vi "Setup Power Supply.vi"(0 "reference in":refnum<class "Power Supply.lvclass">, 1 "Power Supply Chain VISA Session":refnum<visa-resource-name>, 4 "Power Supply Chain Address":i16, 5 "error in (no error)":errorcluster) -> (14 "reference out":refnum<class "Power Supply.lvclass">, 15 "Power Supply Chain VISA Session OUT":refnum<visa-resource-name>, 19 "error out":errorcluster)   [LabVIEW 2017, in "Power Supply.lvclass"]
uses:
  Power Supply.lvclass
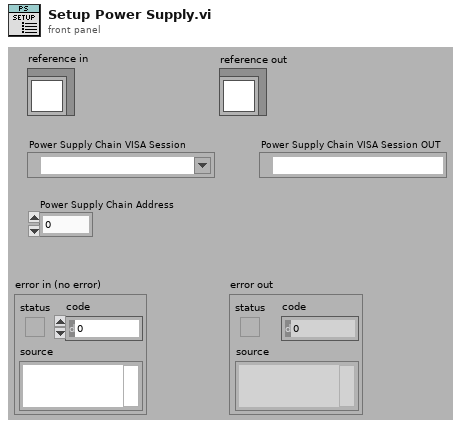
[diagram p1: front panel]
types:
  T1 = typedef "Power Supply.lvclass/ObjectAttributes.ctl" = cluster{"Power Supply Chain VISA Session":refnum<visa-resource-name>, "Power Supply Chain Address":i16, "Power Supply Open/Close Status":bool, "Power Supply Voltage Setting":dbl, "Power Supply Current Setting":dbl, "Power Supply Voltage Reading":dbl, "Power Supply Current Reading":dbl, "Power Supply Status":T2, "Power Supply Error":T3, "Fault Register":u8, "Power Supply Error":bool}
  T2 = typedef "Power Supply.lvclass/Power Supply Status.ctl" = enum16{"Closed", "Open"}
  T3 = typedef "Power Supply.lvclass/Power Supply Error.ctl" = enum16{"None", "Read Error"}
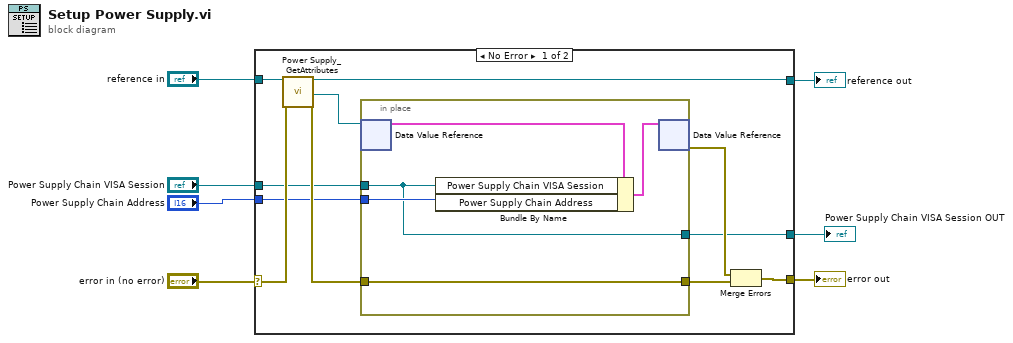
[diagram p0: block diagram]
diagram:
  n1 = case shown="No Error" "error in (no error)" {
    selector: "error in (no error)" -> [w17 w25]
    tunnel: [w14 w25] -> w6
    tunnel: [w15 w24] -> w4
    tunnel: "reference in" -> [w18 w24]
    tunnel: "Power Supply Chain Address" -> [w10 _]
    tunnel: "Power Supply Chain VISA Session" -> [w9 _]
    tunnel: [w8 _] -> w1
    frame No Error {
      n2 = call "Power Supply_GetAttributes.vi"("reference in"=w18, "error in (no error)"=w17) -> ("reference out"=w15:refnum<class "Power Supply.lvclass">, "DataRef"=w13:refnum<data-value>, "error out"=w12:errorcluster)  [unwired: 14 in, 1 out]
      n3 = in-place {
        in-place-border: w12 -> [w21]
        in-place-border: [w21] -> w11
        in-place-border: w10 -> [w20]
        in-place-border: w9 -> [w19]
        in-place-border: [w19] -> w8
        n4 = in-place-dvr #1(w13) -> (w22:T1)  [unwired: 1 out]
        n5 = Bundle By Name(cluster=w22, "Power Supply Chain VISA Session"=w19, "Power Supply Chain Address"=w20) -> (w23:T1)
        n6 = in-place-dvr #1(w23) -> (w16:errorcluster)  [unwired: 1 out]
      }
      n7 = Merge Errors(w16, w11) -> (w14:errorcluster)
    }
    frame Error {
    }
  }
  "error out" <- w6
  "reference out" <- w4
  "Power Supply Chain VISA Session OUT" <- w1
